vi "Password Authentication.vi"(8 "Error In":errorcluster, 9 "Password":string, 10 "Username":string, 11 "Session In":refnum<class "Session.lvclass">) -> (0 "Error Out":errorcluster, 3 "Sesssion Out":refnum<class "Session.lvclass">)   [LabVIEW 2018, in "Toolkit.lvlib" / "Session.lvclass"]
doc: "Authenticates the session using a username and password. This is considered the least secure method of authentication."
uses:
  Session.lvclass
  Session.lvclass/Session.ctl
  SSH/SSH.lvclass/SSH.ctl
  Toolkit.lvlib
  SSH/SSH.lvclass
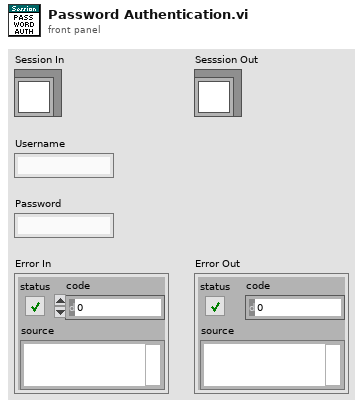
[diagram p1: front panel]
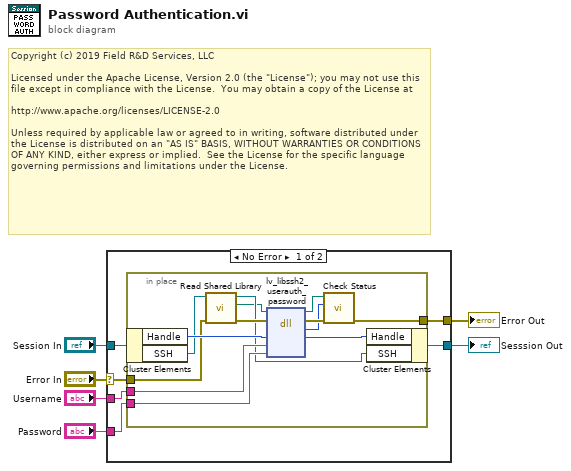
[diagram p0: block diagram]
diagram:
  # "Copyright (c) 2019 Field R&D Services, LLC\n\nLicensed under the Apache License, Version 2.0 (the \"License\"); you may not use this file except in compliance with the License.  You may obtain a copy of the License at\n\nhttp://www.apache.org/licenses/LICENSE-2.0\n\nUnless required by applicable law or agreed to in writing, software distributed under the License is distributed on an \"AS IS\" BASIS, WITHOUT WARRANTIES OR CONDITIONS OF ANY KIND, either express or implied.  See the License for the specific language governing permissions and limitations under the License."
  n1 = case shown="No Error" "Error In" {
    selector: "Error In" -> [w9 w27]
    tunnel: [w11 w27] -> w5
    tunnel: "Session In" -> [w10 w26]
    tunnel: [w12 w26] -> w3
    tunnel: "Username" -> [w8 _]
    tunnel: "Password" -> [w7 _]
    frame No Error {
      n2 = in-place {
        in-place-border: [w23] -> w11
        in-place-border: w9 -> [w19]
        in-place-border: w8 -> [w18]
        in-place-border: w7 -> [w17]
        n3 = in-place-cluster #1(w10) -> ("Handle"=w22:u64, "SSH"=w15:refnum<class "SSH.lvclass">)
        n4 = call "Read Shared Library.vi"("Error In"=w19, "SSH In"=w15) -> ("Error Out"=w16:errorcluster, "libssh2lv Shared Library"=w13:path, "SSH Out"=w14:refnum<class "SSH.lvclass">)  [unwired: 7 in]
        n5 = dll-call lib="D:/Users/cfield/Code/Field R&D Services/SSH/LV-LIBSSH2/LabVIEW/trunk/src/Toolkit/Support/lv-libssh2.*" fn="lv_libssh2_userauth_password"(path in=w13, error in=w16, "session"=w22, "username"=w18, "password"=w17) -> (path out=w25:path, error out=w24:errorcluster, "result"=w20:i32, "session"=w21:u64)  [unwired: 3 in]
        n6 = call "Check Status.vi"("Error In"=w24, "Status"=w20, "libssh2lv Shared Library In"=w25) -> ("Error Out"=w23:errorcluster)  [unwired: 7 in, 1 out]
        n7 = in-place-cluster #1("Handle"=w21, "SSH"=w14) -> (w12:refnum<class "Session.lvclass">)
      }
    }
    frame Error {
    }
  }
  "Sesssion Out" <- w3
  "Error Out" <- w5
